vi "data_transform subVI.vi"(5 "data":dbl[][](array[numeric]), 11 "error in (no error)":errorcluster) -> (4 "Data":dbl[](array[numeric]), 15 "error out":errorcluster)   [LabVIEW 2024]
uses:
  <vilib>/Analysis/2dsp.llb/Real FFT.vi
  <vilib>/Analysis/5stat.llb/RMS (DBL).vi
  <vilib>/Analysis/NI_AALBase.lvlib
  <vilib>/Analysis/NI_AALPro.lvlib
  <vilib>/gmath/NI_Gmath.lvlib
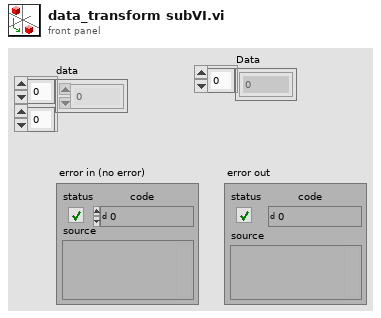
[diagram p1: front panel]
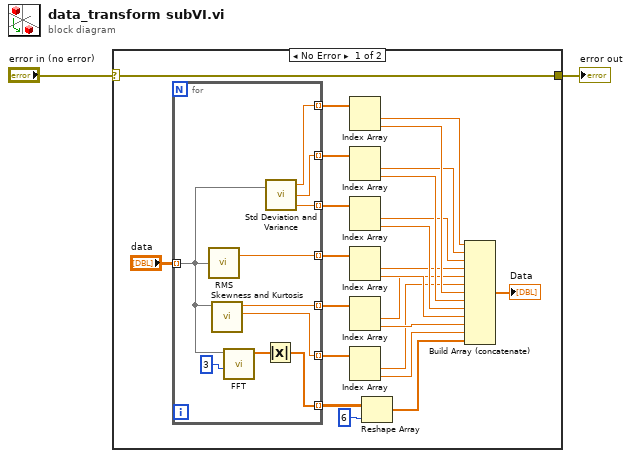
[diagram p0: block diagram]
diagram:
  n1 = case shown="No Error" "error in (no error)" {
    selector: "error in (no error)" -> [w7 w37]
    tunnel: [w7 w37] -> w1
    frame No Error {
      n2 = for {
        tunnel: "data" -> [w28] mode=indexing
        tunnel: [w36] -> w18 mode=indexing
        tunnel: [w35] -> w17 mode=indexing
        tunnel: [w34] -> w16 mode=indexing
        tunnel: [w33] -> w13 mode=indexing
        tunnel: [w32] -> w11 mode=indexing
        tunnel: [w31] -> w9 mode=indexing
        tunnel: [w27] -> w6 mode=indexing
        n3 = call-poly <vilib>:"RMS.vi"("X"=w28) -> ("rms value"=w34:dbl)  [unwired: 1 out]
        n4 = call <vilib>:"Skewness and Kurtosis.vi"("X"=w28) -> ("kurtosis"=w36:dbl, "skewness"=w35:dbl)  [unwired: 8 in, 1 out]
        n5 = call-poly <vilib>:"FFT.vi"("FFT size"=3, "X"=w28) -> ("FFT {X}"=w29:cdb[])  [unwired: 8 in, 1 out]
        n6 = Absolute Value(x=w29) -> (abs(x)=w27:dbl[])
        n7 = call <vilib>:"Std Deviation and Variance.vi"("X"=w28) -> ("mean"=w31:dbl, "standard deviation"=w32:dbl, "variance"=w33:dbl)  [unwired: 1 in]
      }
      n8 = Index Array(array=w9) -> (element #1=w10:dbl, element #2=w21:dbl)  [unwired: 2 in]
      n9 = Index Array(array=w11) -> (element #1=w12:dbl, element #2=w22:dbl)  [unwired: 2 in]
      n10 = Index Array(array=w13) -> (element #1=w14:dbl, element #2=w23:dbl)  [unwired: 2 in]
      n11 = Index Array(array=w16) -> (element #1=w15:dbl, element #2=w24:dbl)  [unwired: 2 in]
      n12 = Index Array(array=w17) -> (element #1=w19:dbl, element #2=w25:dbl)  [unwired: 2 in]
      n13 = Index Array(array=w18) -> (element #1=w20:dbl, element #2=w26:dbl)  [unwired: 2 in]
      n14 = Reshape Array(w6, 6 ("dimension size")) -> (w5:dbl[])
      n15 = Build Array (concatenate)(w10, w12, w14, w15, w19, w20, w21, w22, w23, w24, w25, w26, w5) -> (→"Data":dbl[])
    }
    frame Error {
    }
  }
  "error out" <- w1
